vi "CAN_Send Diag Message.vi"(0 "Write Session in":refnum<k21>, 1 "Enum":T2=enum."Get Calibration Status", 2 "Postion":u16=3, 4 "ECU Info in":T1, 5 "Read Session in":refnum<k21>, 7 "ODX File Path":path=path "C:/LegacyApp/DB_0CA_7100_4M0_0004_73710BVW3710/DB_0CA_7100_4M0_0004_73710BVW3710/DB_0CA_7100_4M0_0004_73710BVW3710.odx", 8 "Tester":refnum<k21>, 9 "Tx Msg":u8[](array[numeric])=[2, 26, 156, 255, 255, 255, 255, 255] format="%02x", 11 "error in (no error)":errorcluster, 12 "Download CAL Progress":refnum<vi>, 13 "Download CAL Time":refnum<vi>) -> (6 "ECU Info":T1, 10 "TxRx Data":string[][](array[string]), 14 "Response Good?":bool, 15 "error out":errorcluster)   [LabVIEW 2014]
uses:
  Diagnostic Message.ctl
  <vilib>/xnet/xnet.llb/XNET Frame CAN.ctl
  <vilib>/xnet/xnet.llb/XNET Frame Type CAN.ctl
  CAN Communication VI's/Typedefs/Select Session.ctl
  typedefs/All Motions.ctl
  <vilib>/xnet/xnet.llb/XNET Write (Frame CAN).vi
  <vilib>/xnet/xnet.llb/XNET Read (Frame CAN).vi
panel:
  out "Rx Message":u8[](array[numeric]) format="%02x"
  out "Error String Out":string
  in  "Tx Arbitration Id":u32=402391172 format="%.0x"
  out "Part Number":string
  out "Vehicle Type":string
  out "SW level":string
  out "Calibrated":bool
  out "HW level":string
  out "CAL level":string
  out "Boot level":string
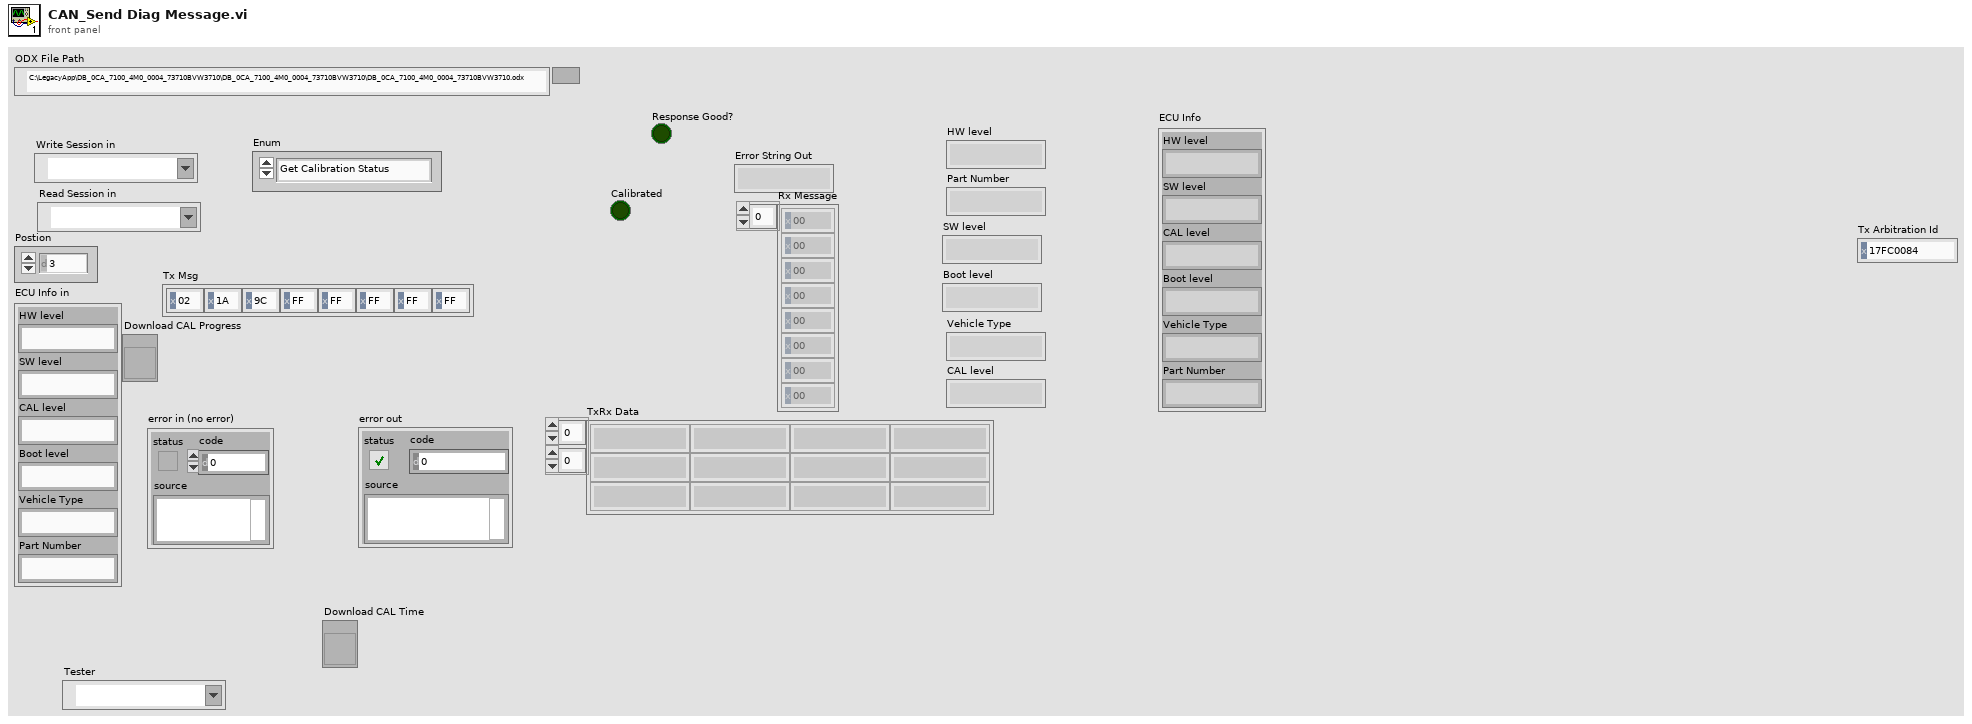
[diagram p1: front panel]
types:
  T1 = cluster{"HW level":string, "SW level":string, "CAL level":string, "Boot level":string, "Vehicle Type":string, "Part Number":string}
  T2 = typedef "Diagnostic Message.ctl" = enum16{"User Select", "Get User Multi-Frame", "Diag Session Prog", "Diag Session Ext", "Diag Session EOL", "Diag Session Default", "Diag Session Dev", "Read Active Session", "Read HW", "Read SW", "Read Part Number", "Learn Start Glass", "Learn Start Rollo", "Get Calibration Status", "Read SW CAL Boot", "Go to Position", "Get Parametric Mode Status", "Enable Parametric Mode", "Disable Parametric Mode", "Enable Production Mode", "Disable Production Mode", "Reset ECU", "Go to Slide Close", "Go to Slide Open", "Go to Vent Open", "Rollo Open", "Rollo Close", "Write Vehicle Type", "Read Vehicle Type", "Clear DTC", "Check Teach DTC", "Write Shop Code", "Download CAL"}
  T3 = typedef "XNET Frame CAN.ctl" = cluster{"timestamp":timestamp, "payload":u8[], "identifier":u32, "type":T4, "extended?":bool, "echo?":bool}
  T4 = typedef "XNET Frame Type CAN.ctl" = u8
  T5 = typedef "Select Session.ctl" = enum16{"DefaultSession", "Development", "Extended", "EOL", "Programming"}
  T6 = typedef "All Motions.ctl" = enum16{"Idle", "Glass Teach", "Glass Slide Open", "Glass Slide Open 2", "Glass Slide Close", "Glass Slide Close 2", "Glass Vent Open", "Glass Vent Close", "Sunshade Teach", "Sunshade Teach 2", "Sunshade Open", "Sunshade Open 2", "Sunshade Close", "Sunshade Close 2", "Glass Slide Open Sunshade Open", "Glass Slide Open 2 Sunshade Open", "Glass Slide Open Sunshade Close", "Glass Slide Open 2 Sunshade Close", "Glass Slide Close Sunshade Open", "Glass Slide Close 2 Sunshade Open", "Glass Slide Close Sunshade Close", "Glass Slide Close 2 Sunshade Close", "Glass Vent Open Sunshade Open", "Glass Vent Open Sunshade Close", "Glass Vent Close Sunshade Open", "Glass Vent Close Sunshade Close", "Express Glass Slide Open", "Express Glass Slide Open 2", "Express Glass Slide Close", "Express Glass Slide Close 2", "Express Glass Vent Open", "Express Glass Vent Close", "Express Sunshade Open", "Express Sunshade Close", "Express Sunshade Open 2", "Express Sunshade Close 2", "Express Glass Slide Open Sunshade Open", "Express Glass Slide Open 2 Sunshade Open", "Express Glass Slide Open Sunshade Close", "Express Glass Slide Open 2 Sunshade Close", "Express Glass Slide Close Sunshade Open", "Express Glass Slide Close 2 Sunshade Open", "Express Glass Slide Close Sunshade Close", "Express Glass Slide Close 2 Sunshade Close", "Express Glass Vent Open Sunshade Open", "Express Glass Vent Open Sunshade Close", "Express Glass Vent Close Sunshade Open", "Express Glass Vent Close Sunshade Close", "Goto Position Glass", "Goto Position Sunshade"}
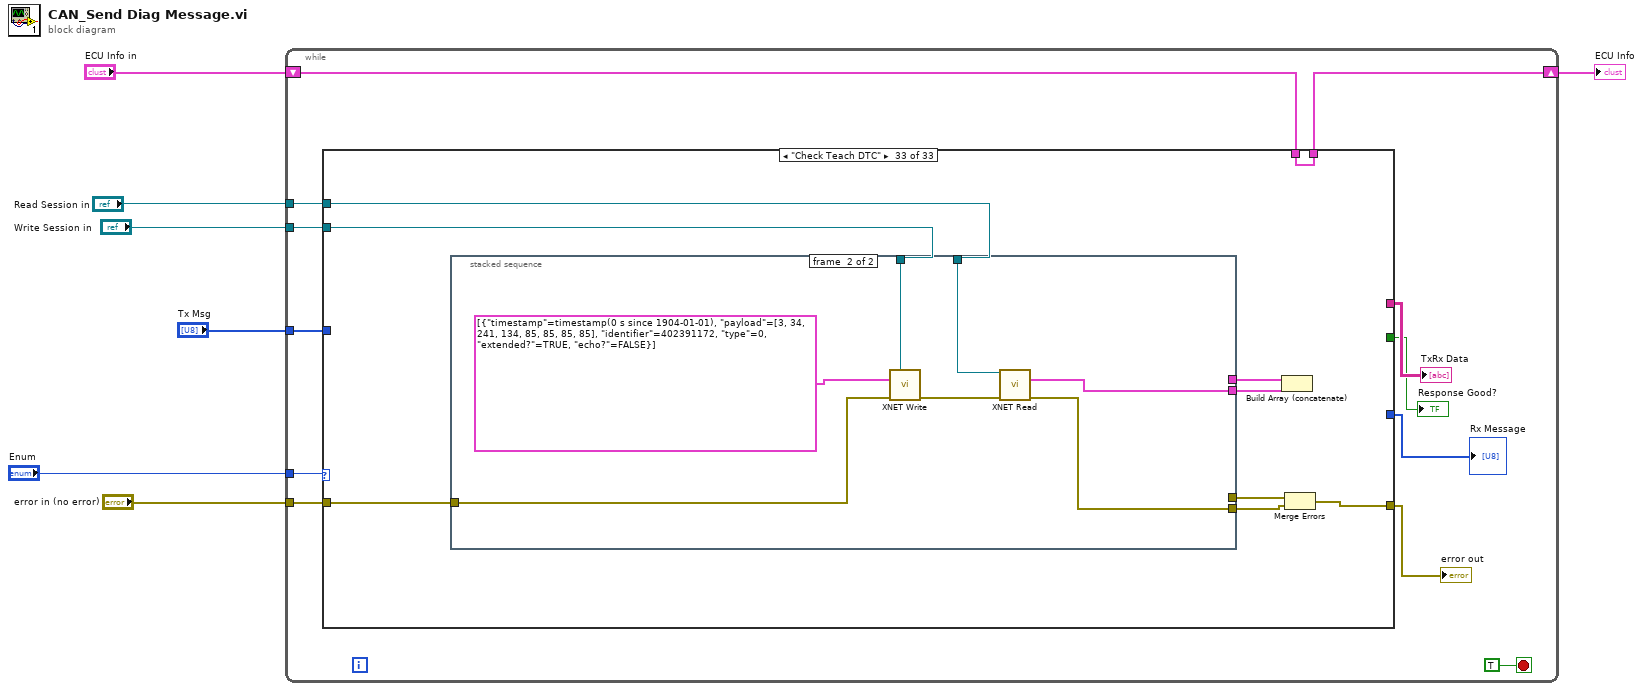
[diagram p0: block diagram]
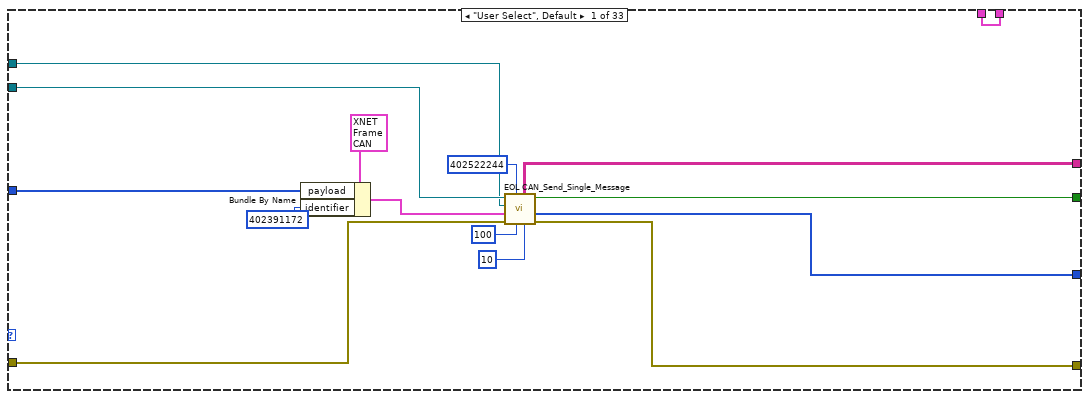
[diagram p2: hidden frame]
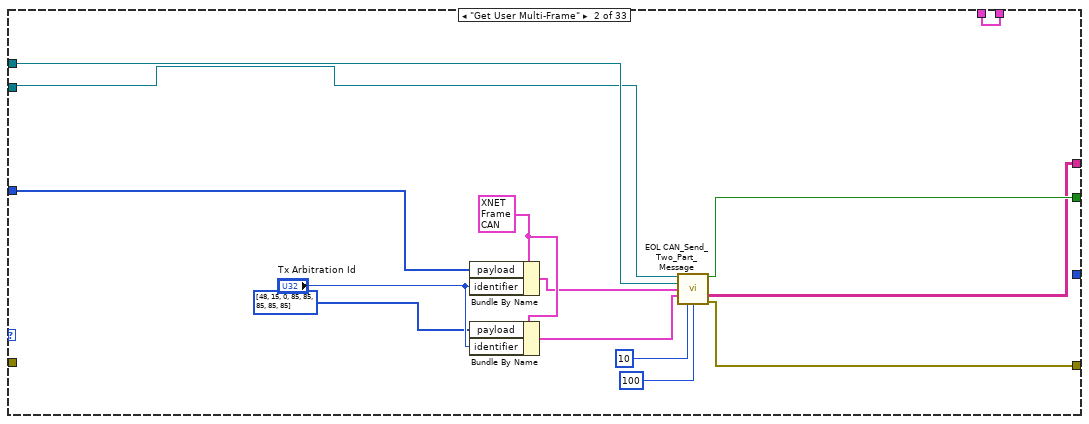
[diagram p3: hidden frame]
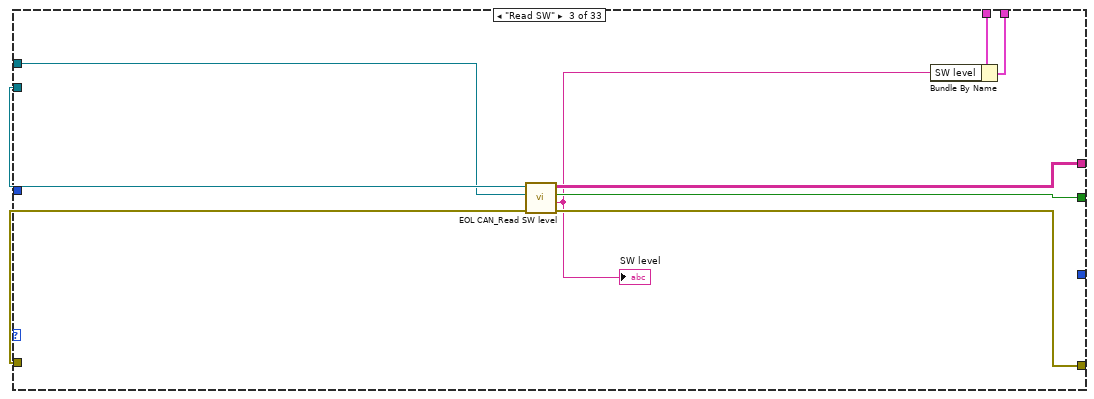
[diagram p4: hidden frame]
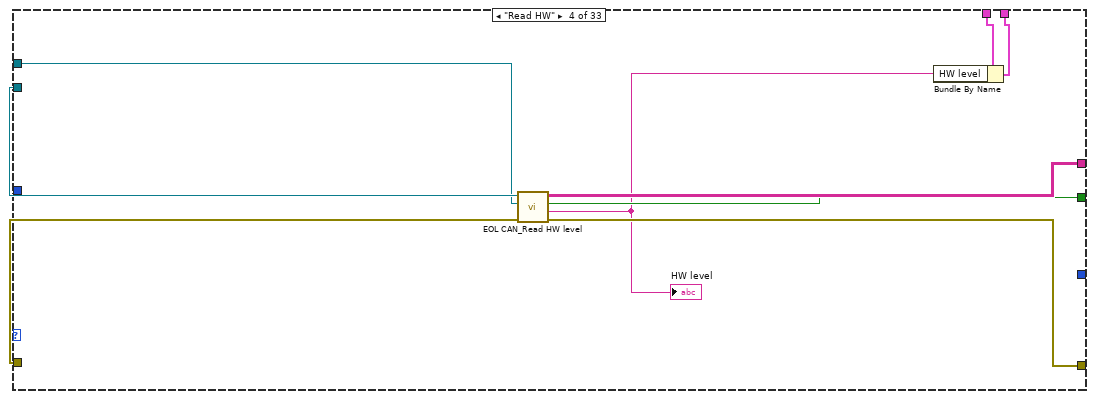
[diagram p5: hidden frame]
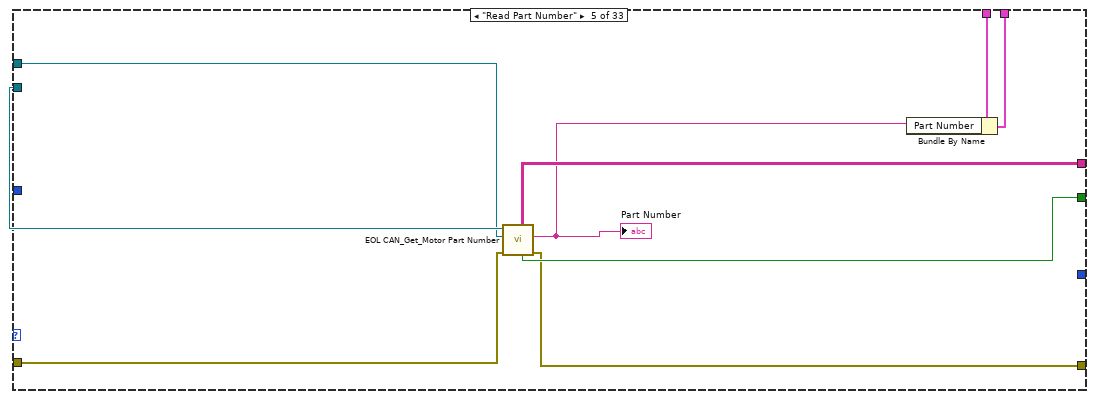
[diagram p6: hidden frame]
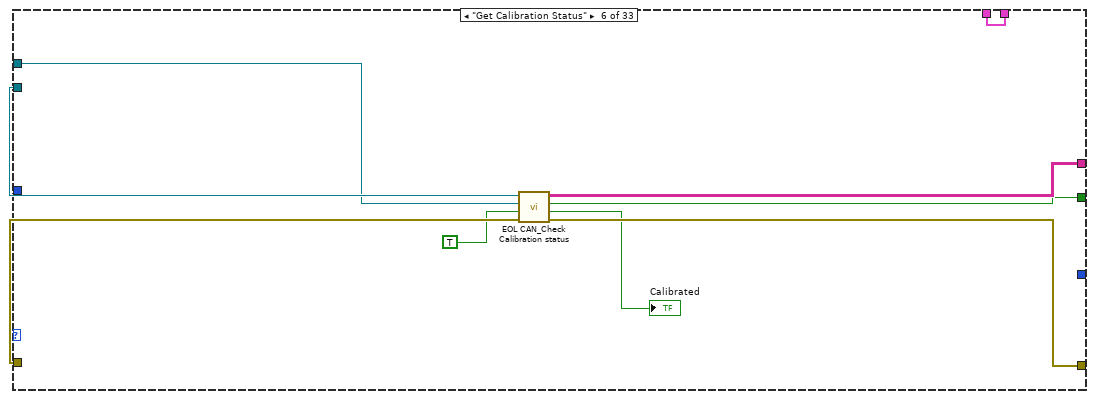
[diagram p7: hidden frame]
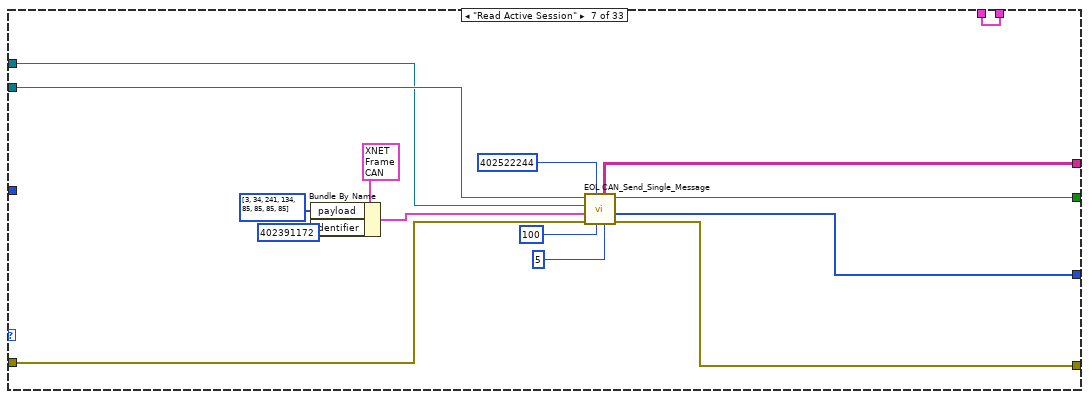
[diagram p8: hidden frame]
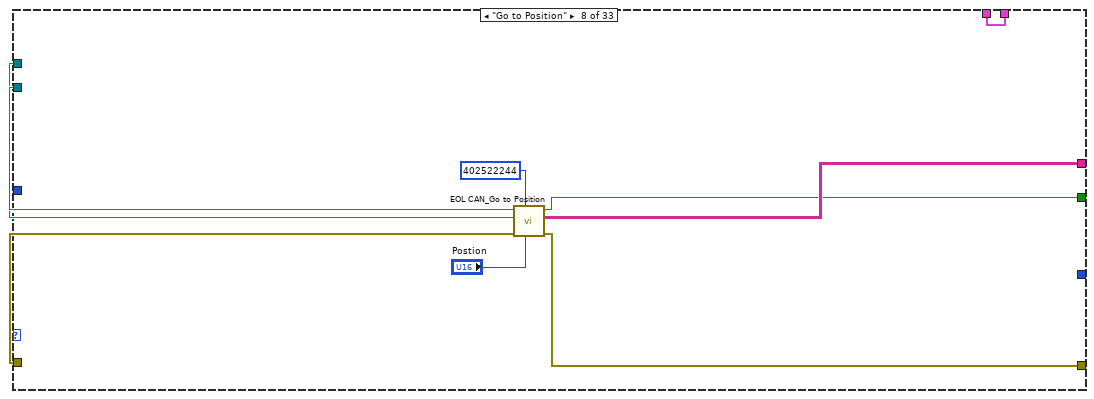
[diagram p9: hidden frame]
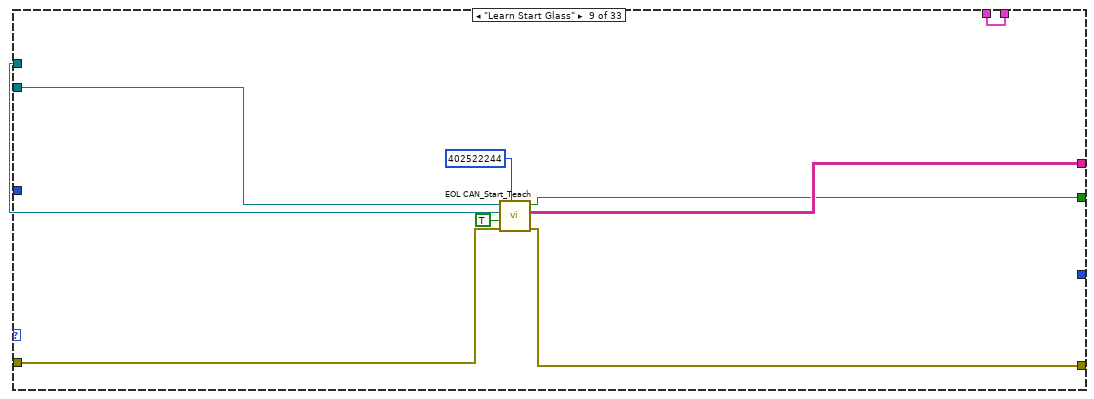
[diagram p10: hidden frame]
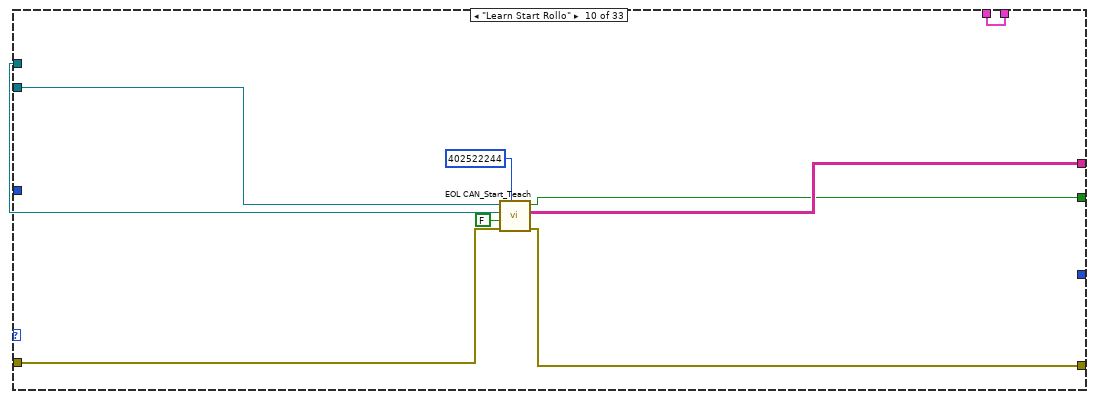
[diagram p11: hidden frame]
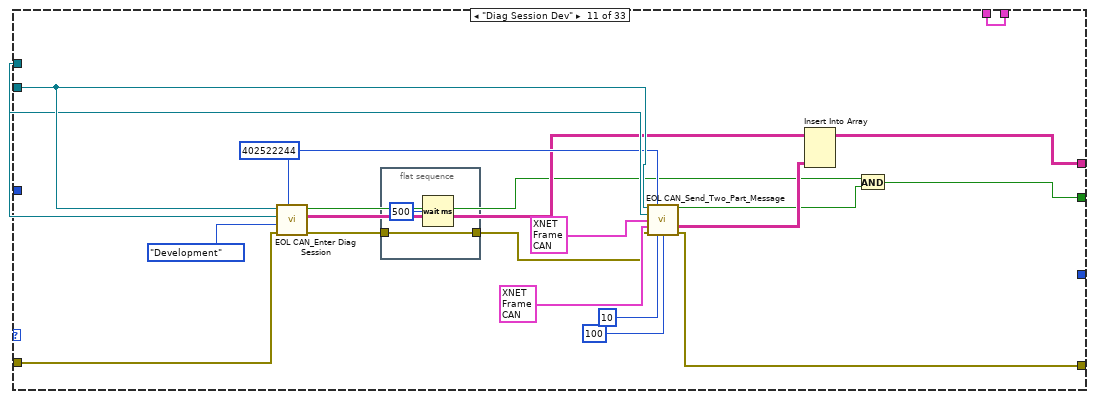
[diagram p12: hidden frame]
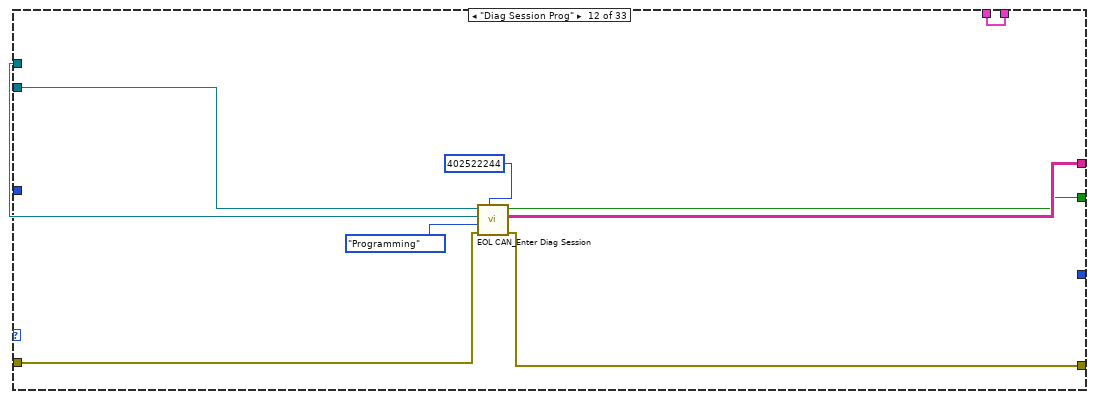
[diagram p13: hidden frame]
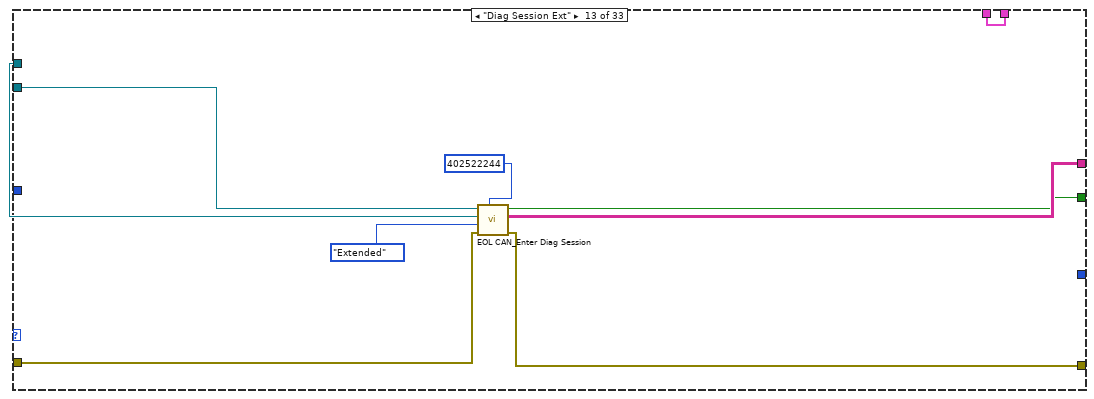
[diagram p14: hidden frame]
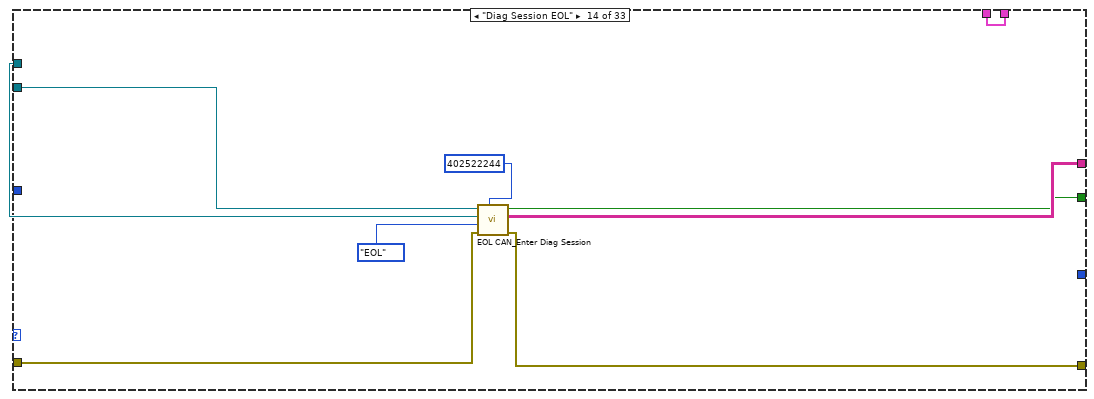
[diagram p15: hidden frame]
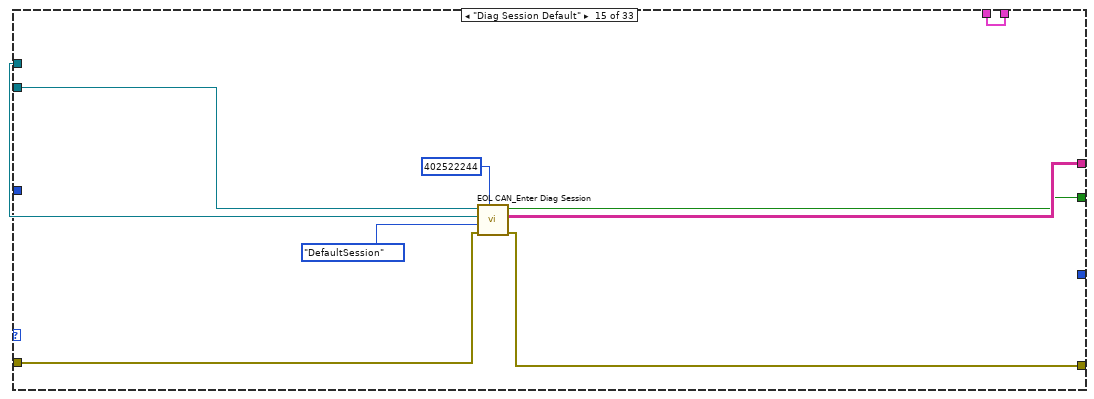
[diagram p16: hidden frame]
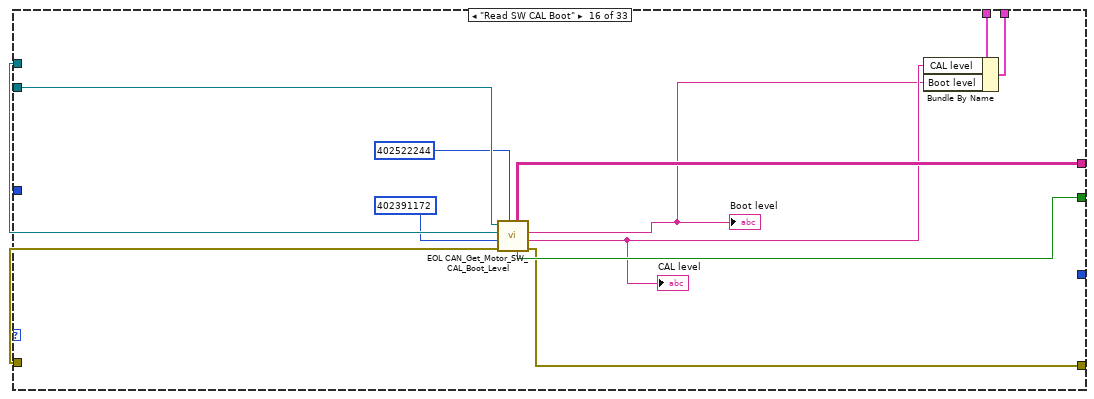
[diagram p17: hidden frame]
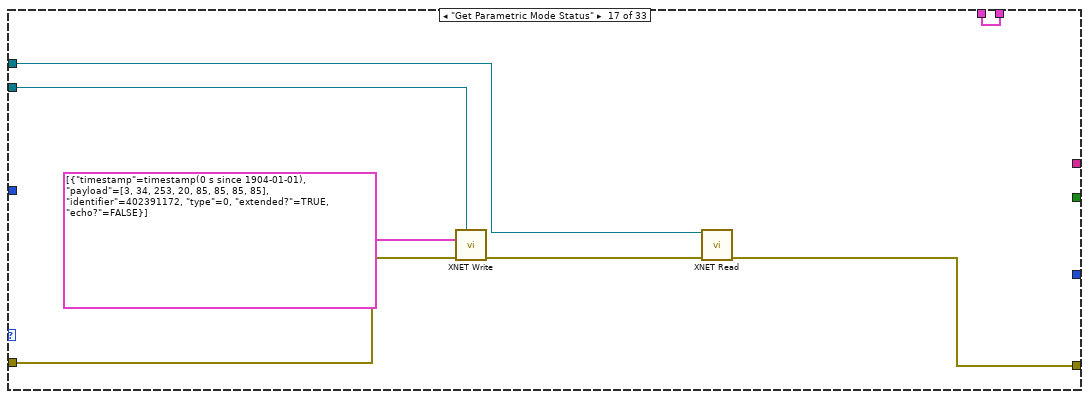
[diagram p18: hidden frame]
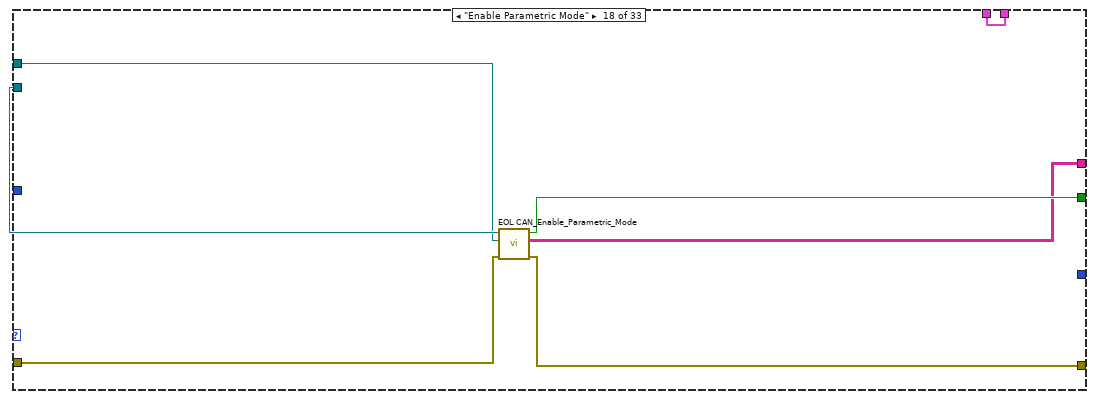
[diagram p19: hidden frame]
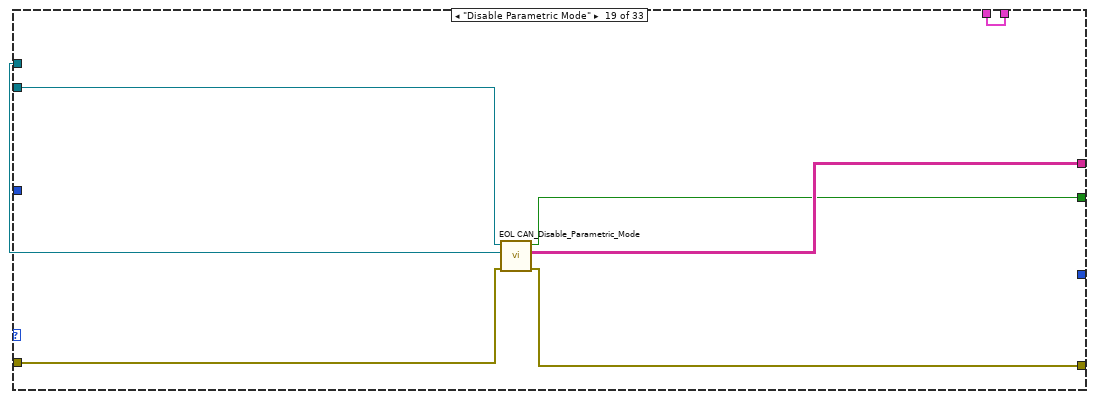
[diagram p20: hidden frame]
diagram:
  n1 = while {
    tunnel: "error in (no error)" -> [w19]
    tunnel: "Read Session in" -> [w17]
    tunnel: "Write Session in" -> [w16]
    tunnel: "Enum" -> [w15]
    shift-right: [w11] -> w3
    shift-left: "ECU Info in" -> [w10]
    tunnel: "Tx Msg" -> [w9]
    stop <- TRUE stop-if-true
    n2 = case shown="\"Check Teach DTC\"" w15 {
      tunnel: w17 -> [w33 w40 w52 w61 w73 w83 w98 w105 w115 w124 w141 w150 w159 w168 w177 w193 w200 w207 w211 w221 w228 w236 w245 w254 w263 w272 w281 w284 w291 w305 w319 w325 w334]
      tunnel: w16 -> [w34 w39 w53 w62 w74 w84 w99 w106 w116 w125 w143 w151 w160 w169 w178 w194 w202 w208 w212 w222 w229 w237 w246 w255 w264 w273 w282 w285 w292 w306 w318 w326 w336]
      tunnel: w19 -> [w32 _ w57 w66 w75 w82 w97 w108 w117 w126 w145 w156 w165 w174 w183 w195 w201 w209 w216 w223 w230 w238 w247 w256 w265 w274 w283 _ _ _ w320 w327 w335]
      tunnel: [w31 w35 w56 w65 w70 w81 w96 w107 w113 w122 w142 w155 w164 w173 w182 w188 w197 w204 w215 w218 w225 w232 w241 w250 w259 w268 w277 w288 w295 errorcluster {"status"=FALSE, "code"=0, "source"=""} ("error IO") w313 w324 w333] -> w18
      tunnel: [w30 w36 w55 w64 w72 w80 w95 w103 w112 w121 w135 w154 w163 w172 w181 w190 _ w205 w214 w219 w226 w234 w242 w251 w260 w269 w278 w289 w296 w301 w315 w322 _] -> w14
      tunnel: [w29 w37 w54 w63 w71 w77 w94 w102 w111 w120 w132 w153 w162 w171 w180 w189 _ w206 w213 w220 w227 w233 w243 w252 w261 w270 w279 w287 w294 w298 w314 w323 _] -> w13
      tunnel: [w28 _ _ _ _ _ w91 _ _ _ _ _ _ _ _ _ _ _ _ _ _ _ _ _ _ _ _ w286 w293 _ _ _ _] -> w8
      tunnel: [w21 w48 w50 w58 w68 w76 w85 w100 w110 w119 w127 w148 w157 w166 w175 w186 w196 w203 w210 w217 w224 w231 w239 w248 w257 w266 w275 w290 w297 w309 w311 w321 w328] -> w11
      tunnel: w10 -> [w21 w48 w51 w59 w67 w76 w85 w100 w110 w119 w127 w148 w157 w166 w175 w187 w196 w203 w210 w217 w224 w231 w239 w248 w257 w266 w275 w290 w297 w309 w312 w321 w328]
      tunnel: w9 -> [w20 w38 _ _ _ _ _ _ _ _ _ _ _ _ _ _ _ _ _ _ _ _ _ _ _ _ _ _ _ _ _ _ _]
      frame "User Select", Default {
        n3 = Bundle By Name(cluster=T3 {"timestamp"=timestamp(0 s since 1904-01-01), "payload"=[2, 39, 3, 85, 85, 85, 85, 85], "identifier"=402391172, "type"=0, "extended?"=TRUE, "echo?"=FALSE} ("Tx CAN frame"), "payload"=w20, "identifier"=u32 402391172) -> (w26:T3)
        n4 = call "EOL CAN_Send_Single_Message.vi"("Retries"=10, "Msg Wait Time"=u32 100, "Rx Arbitration Id"=u32 402522244, "Error in"=w32, "Tx CAN frame"=w26, "Read Session in"=w33, "Write Session in"=w34) -> ("Error out"=w31:errorcluster, "Rx Message"=w28:u8[], "Response Good?"=w29:bool, "TxRx Data"=w30:string[][])  [unwired: 1 out]
      }
      frame "Get User Multi-Frame" {
        w42 = T3 {"timestamp"=timestamp(0 s since 1904-01-01), "payload"=[2, 39, 3, 85, 85, 85, 85, 85], "identifier"=402391172, "type"=0, "extended?"=TRUE, "echo?"=FALSE} ("Tx CAN frame 1")
        n5 = Bundle By Name(cluster=w42, "payload"=w38, "identifier"="Tx Arbitration Id") -> (w41:T3)
        n6 = Bundle By Name(cluster=w42, "payload"=u8[] [48, 15, 0, 85, 85, 85, 85, 85] ("Transmit Data"), "identifier"="Tx Arbitration Id") -> (w43:T3)
        n7 = call "EOL CAN_Send_Two_Part_Message.vi"("Write Session in"=w39, "Read Session in"=w40, "Tx CAN frame 1"=w41, "Tx CAN frame 2"=w43, "Retries"=10, "Msg Wait Time"=u32 100) -> ("Response Good?"=w37:bool, "TxRx Data"=w36:string[][], "error out"=w35:errorcluster)  [unwired: 6 in, 1 out]
      }
      frame "Read SW" {
        n8 = call "EOL CAN_Read SW level.vi"("error in (no error)"=w57, "Read Session in"=w52, "Write Session in"=w53) -> ("error out"=w56:errorcluster, "SW level"=w49:string, "Response Good?"=w54:bool, "TxRx Data"=w55:string[][])  [unwired: 5 in]
        "SW level" <- w49
        n9 = Bundle By Name(cluster=w51, "SW level"=w49) -> (w50:T1)
      }
      frame "Read HW" {
        n10 = call "EOL CAN_Read HW level.vi"("error in (no error)"=w66, "Read Session in"=w61, "Write Session in"=w62) -> ("error out"=w65:errorcluster, "HW level"=w60:string, "Response Good?"=w63:bool, "TxRx Data"=w64:string[][])  [unwired: 5 in]
        "HW level" <- w60
        n11 = Bundle By Name(cluster=w59, "HW level"=w60) -> (w58:T1)
      }
      frame "Read Part Number" {
        n12 = call "EOL CAN_Get_Motor Part Number.vi"("error in (no error)"=w75, "Read Session in"=w73, "Write Session in"=w74) -> ("error out"=w70:errorcluster, "Part Number"=w69:string, "Response Good?"=w71:bool, "TxRx Data"=w72:string[][])  [unwired: 5 in]
        "Part Number" <- w69
        n13 = Bundle By Name(cluster=w67, "Part Number"=w69) -> (w68:T1)
      }
      frame "Get Calibration Status" {
        n14 = call "EOL CAN_Check Calibration status.vi"("error in (no error)"=w82, "Glass?"=TRUE, "Read Session in"=w83, "Write Session in"=w84) -> ("error out"=w81:errorcluster, "Calibrated"=→"Calibrated":bool, "Response Good?"=w77:bool, "TxRx Data"=w80:string[][])  [unwired: 4 in]
      }
      frame "Read Active Session" {
        n15 = Bundle By Name(cluster=T3 {"timestamp"=timestamp(0 s since 1904-01-01), "payload"=[2, 39, 3, 85, 85, 85, 85, 85], "identifier"=402391172, "type"=0, "extended?"=TRUE, "echo?"=FALSE} ("Tx CAN frame"), "payload"=u8[] [3, 34, 241, 134, 85, 85, 85, 85], "identifier"=u32 402391172) -> (w88:T3)
        n16 = call "EOL CAN_Send_Single_Message.vi"("Retries"=5, "Msg Wait Time"=u32 100, "Rx Arbitration Id"=u32 402522244, "Error in"=w97, "Tx CAN frame"=w88, "Read Session in"=w98, "Write Session in"=w99) -> ("Error out"=w96:errorcluster, "Rx Message"=w91:u8[], "Response Good?"=w94:bool, "TxRx Data"=w95:string[][])  [unwired: 1 out]
      }
      frame "Go to Position" {
        n17 = call "EOL CAN_Go to Position.vi"("Postion"="Postion", "Rx Arbitration Id"=u32 402522244, "Error in"=w108, "Read Session in"=w105, "Write Session in"=w106) -> ("Error out"=w107:errorcluster, "TxRx Data"=w103:string[][], "Response Good?"=w102:bool)  [unwired: 4 in]
      }
      frame "Learn Start Glass" {
        n18 = call "EOL CAN_Start_Teach.vi"("Rx Arbitration Id"=u32 402522244, "Error in"=w117, "Glass?"=TRUE, "Read Session in"=w115, "Write Session in"=w116) -> ("Error out"=w113:errorcluster, "TxRx Data"=w112:string[][], "Response Good?"=w111:bool)  [unwired: 4 in]
      }
      frame "Learn Start Rollo" {
        n19 = call "EOL CAN_Start_Teach.vi"("Rx Arbitration Id"=u32 402522244, "Error in"=w126, "Glass?"=FALSE, "Read Session in"=w124, "Write Session in"=w125) -> ("Error out"=w122:errorcluster, "TxRx Data"=w121:string[][], "Response Good?"=w120:bool)  [unwired: 4 in]
      }
      frame "Diag Session Dev" {
        w140 = u32 402522244 ("Rx Arbitration Id")
        n20 = call "EOL CAN_Enter Diag Session.vi"("Rx Arbitration Id"=w140, "Error in"=w145, "Session"=Select_Session."Development", "Read Session in"=w141, "Write Session in"=w143) -> ("Error out"=w131:errorcluster, "TxRx Data"=w137:string[][], "Response Good?"=w133:bool)  [unwired: 4 in]
        n21 = flat-sequence {
          tunnel: w131 -> [w146]
          tunnel: [w146] -> w130
          frame #0 {
            n22 = Wait (ms)(milliseconds to wait=u32 500) -> ()  [unwired: 1 out]
          }
        }
        n23 = call "EOL CAN_Send_Two_Part_Message.vi"("Write Session in"=w143, "Rx Arbitration Id"=w140, "Read Session in"=w141, "Tx CAN frame 1"=T3 {"timestamp"=timestamp(0 s since 1904-01-01), "payload"=[3, 34, 254, 253, 85, 85, 85, 85], "identifier"=402391172, "type"=8, "extended?"=TRUE, "echo?"=FALSE}, "Tx CAN frame 2"=T3 {"timestamp"=timestamp(0 s since 1904-01-01), "payload"=[48, 15, 0, 85, 85, 85, 85, 85], "identifier"=402391172, "type"=8, "extended?"=TRUE, "echo?"=FALSE}, "error in (no error)"=w130, "Retries"=10, "Msg Wait Time"=u32 100) -> ("Response Good?"=w134:bool, "TxRx Data"=w136:string[][], "error out"=w142:errorcluster)  [unwired: 4 in, 1 out]
        n24 = Insert Into Array(array=w137, new element=w136) -> (w135:string[][])  [unwired: 2 in]
        n25 = And(x=w133, y=w134) -> (x .and. y?=w132:bool)
      }
      frame "Diag Session Prog" {
        n26 = call "EOL CAN_Enter Diag Session.vi"("Rx Arbitration Id"=u32 402522244, "Error in"=w156, "Session"=Select_Session."Programming", "Read Session in"=w150, "Write Session in"=w151) -> ("Error out"=w155:errorcluster, "TxRx Data"=w154:string[][], "Response Good?"=w153:bool)  [unwired: 4 in]
      }
      frame "Diag Session Ext" {
        n27 = call "EOL CAN_Enter Diag Session.vi"("Rx Arbitration Id"=u32 402522244, "Error in"=w165, "Session"=Select_Session."Extended", "Read Session in"=w159, "Write Session in"=w160) -> ("Error out"=w164:errorcluster, "TxRx Data"=w163:string[][], "Response Good?"=w162:bool)  [unwired: 4 in]
      }
      frame "Diag Session EOL" {
        n28 = call "EOL CAN_Enter Diag Session.vi"("Rx Arbitration Id"=u32 402522244, "Error in"=w174, "Session"=Select_Session."EOL", "Read Session in"=w168, "Write Session in"=w169) -> ("Error out"=w173:errorcluster, "TxRx Data"=w172:string[][], "Response Good?"=w171:bool)  [unwired: 4 in]
      }
      frame "Diag Session Default" {
        n29 = call "EOL CAN_Enter Diag Session.vi"("Rx Arbitration Id"=u32 402522244, "Error in"=w183, "Session"=Select_Session."DefaultSession", "Read Session in"=w177, "Write Session in"=w178) -> ("Error out"=w182:errorcluster, "TxRx Data"=w181:string[][], "Response Good?"=w180:bool)  [unwired: 4 in]
      }
      frame "Read SW CAL Boot" {
        n30 = call "EOL CAN_Get_Motor_SW_CAL_Boot_Level.vi"("Rx Arbitration Id"=u32 402522244, "error in (no error)"=w195, "Tx Arbitration Id"=u32 402391172 ("identifier"), "Read Session in"=w193, "Write Session in"=w194) -> ("error out"=w188:errorcluster, "CAL level"=w185:string, "Boot level"=w184:string, "Response Good?"=w189:bool, "TxRx Data"=w190:string[][])  [unwired: 1 in, 1 out]
        "Boot level" <- w184
        "CAL level" <- w185
        n31 = Bundle By Name(cluster=w187, "CAL level"=w185, "Boot level"=w184) -> (w186:T1)
      }
      frame "Get Parametric Mode Status" {
        n32 = call-poly <vilib>:"XNET Write.vi"("session in"=w202, "data"=T3[] [{"timestamp"=timestamp(0 s since 1904-01-01), "payload"=[3, 34, 253, 20, 85, 85, 85, 85], "identifier"=402391172, "type"=0, "extended?"=TRUE, "echo?"=FALSE}] ("Frame to Send 2"), "error in (no error)"=w201) -> ("error out"=w198:errorcluster)  [unwired: 11 in, 1 out]
        n33 = call-poly <vilib>:"XNET Read.vi"("session in"=w200, "error in (no error)"=w198) -> ("error out"=w197:errorcluster)  [unwired: 10 in, 3 out]
      }
      frame "Enable Parametric Mode" {
        n34 = call "EOL CAN_Enable_Parametric_Mode.vi"("Error in"=w209, "Read Session in"=w207, "Write Session in"=w208) -> ("Error out"=w204:errorcluster, "debug log"=w205:string[][], "Response Good?"=w206:bool)  [unwired: 6 in]
      }
      frame "Disable Parametric Mode" {
        n35 = call "EOL CAN_Disable_Parametric_Mode.vi"("Error in"=w216, "Read Session in"=w211, "Write Session in"=w212) -> ("Error out"=w215:errorcluster, "debug log"=w214:string[][], "Response Good?"=w213:bool)  [unwired: 6 in]
      }
      frame "Enable Production Mode" {
        n36 = call "EOL CAN_Enable_Production_Mode.vi"("Error in"=w223, "Read Session in"=w221, "Write Session in"=w222) -> ("Error out"=w218:errorcluster, "debug log"=w219:string[][], "Response Good?"=w220:bool)  [unwired: 6 in]
      }
      frame "Disable Production Mode" {
        n37 = call "EOL CAN_Disable_Production_Mode.vi"("Error in"=w230, "Read Session in"=w228, "Write Session in"=w229) -> ("Error out"=w225:errorcluster, "debug log"=w226:string[][], "Response Good?"=w227:bool)  [unwired: 6 in]
      }
      frame "Reset ECU" {
        n38 = call "EOL CAN_Reset ECU.vi"("Rx Arbitration Id"=u32 402522244, "Error in"=w238, "Read Session in"=w236, "Write Session in"=w237) -> ("Error out"=w232:errorcluster, "Response Good?"=w233:bool, "TxRx Data"=w234:string[][])  [unwired: 5 in]
      }
      frame "Go to Slide Close" {
        n39 = call "EOL CAN_Target Motion.vi"("Rx Arbitration Id"=u32 402522244, "Error in"=w247, "All Motions"=All_Motions."Glass Slide Close", "Read Session in"=w245, "Write Session in"=w246) -> ("Error out"=w241:errorcluster, "TxRx Data"=w242:string[][], "Response Good?"=w243:bool)  [unwired: 4 in]
      }
      frame "Go to Slide Open" {
        n40 = call "EOL CAN_Target Motion.vi"("Rx Arbitration Id"=u32 402522244, "Error in"=w256, "All Motions"=All_Motions."Glass Slide Open", "Read Session in"=w254, "Write Session in"=w255) -> ("Error out"=w250:errorcluster, "TxRx Data"=w251:string[][], "Response Good?"=w252:bool)  [unwired: 4 in]
      }
      frame "Go to Vent Open" {
        n41 = call "EOL CAN_Target Motion.vi"("Rx Arbitration Id"=u32 402522244, "Error in"=w265, "All Motions"=All_Motions."Glass Vent Open", "Read Session in"=w263, "Write Session in"=w264) -> ("Error out"=w259:errorcluster, "TxRx Data"=w260:string[][], "Response Good?"=w261:bool)  [unwired: 4 in]
      }
      frame "Rollo Open" {
        n42 = call "EOL CAN_Target Motion.vi"("Rx Arbitration Id"=u32 402522244, "Error in"=w274, "All Motions"=All_Motions."Sunshade Open", "Read Session in"=w272, "Write Session in"=w273) -> ("Error out"=w268:errorcluster, "TxRx Data"=w269:string[][], "Response Good?"=w270:bool)  [unwired: 4 in]
      }
      frame "Rollo Close" {
        n43 = call "EOL CAN_Target Motion.vi"("Rx Arbitration Id"=u32 402522244, "Error in"=w283, "All Motions"=All_Motions."Sunshade Close", "Read Session in"=w281, "Write Session in"=w282) -> ("Error out"=w277:errorcluster, "TxRx Data"=w278:string[][], "Response Good?"=w279:bool)  [unwired: 4 in]
      }
      frame "Write Vehicle Type" {
        n44 = call "EOL CAN_Write Vehicle Type.vi"("Read Session in"=w284, "Write Session in"=w285) -> ("error out"=w288:errorcluster, "Rx Message"=w286:u8[], "Response Good?"=w287:bool, "Array"=w289:string[][])  [unwired: 6 in]
      }
      frame "Write Shop Code" {
        n45 = call "EOL CAN_Write Repair Shop Code.vi"("Read Session in"=w291, "Write Session in"=w292) -> ("error out"=w295:errorcluster, "Rx Message"=w293:u8[], "Response Good?"=w294:bool, "TxRxData"=w296:string[][])  [unwired: 6 in]
      }
      frame "Download CAL" {
        n46 = call "EOL CAN_Download CAL.vi"("Download CAL Progress"="Download CAL Progress", "Download CAL Time"="Download CAL Time", "ODX File Path"="ODX File Path", "Tester"="Tester", "Glass?"=TRUE, "Read Session in"=w305, "DSC Write Session in"=w306) -> ("Error String Out"=→"Error String Out":string, "TxRx Data"=w301:string[][], "Response Good?"=w298:bool)  [unwired: 2 in]
      }
      frame "Read Vehicle Type" {
        n47 = call "EOL CAN_Get Vehicle type.vi"("Rx Arbitration Id"=u32 402522244, "error in (no error)"=w320, "Tx Arbitration Id"=u32 402391172, "Read Session in"=w319, "Write Session in"=w318) -> ("error out"=w313:errorcluster, "Vehicle Type"=w310:string, "Response Good?"=w314:bool, "TxRx Data"=w315:string[][])  [unwired: 3 in]
        "Vehicle Type" <- w310
        n48 = Bundle By Name(cluster=w312, "Vehicle Type"=w310) -> (w311:T1)
      }
      frame "Clear DTC" {
        n49 = call "EOL CAN_Clear_DTC's.vi"("Error in"=w327, "Read Session in"=w325, "Write Session in"=w326) -> ("Error out"=w324:errorcluster, "TxRx Data"=w322:string[][], "Response Good?"=w323:bool)  [unwired: 6 in]
      }
      frame "Check Teach DTC" {
        n50 = stacked-sequence {
          tunnel: w336 -> [w344 w352]
          tunnel: w335 -> [w343 w351]
          tunnel: [w341 _] -> w332
          tunnel: w334 -> [w342 w350]
          tunnel: [w340 _] -> w330
          tunnel: [_ w349] -> w329
          tunnel: [_ w348] -> w331
          frame #0 {
            n51 = call-poly <vilib>:"XNET Write.vi"("session in"=w344, "data"=T3[] [{"timestamp"=timestamp(0 s since 1904-01-01), "payload"=[2, 16, 79, 85, 85, 85, 85, 85], "identifier"=402391172, "type"=0, "extended?"=TRUE, "echo?"=FALSE}] ("Frame to Send 2"), "error in (no error)"=w343) -> ("error out"=w338:errorcluster)  [unwired: 11 in, 1 out]
            n52 = call "Time Delay22"("error in (no error)"=w338, "Delay Time (s)"=0.05) -> ("error out"=w337:errorcluster)  [unwired: 9 in]
            n53 = call-poly <vilib>:"XNET Read.vi"("session in"=w342, "error in (no error)"=w337) -> ("data"=w340:T3[], "error out"=w341:errorcluster)  [unwired: 10 in, 2 out]
          }
          frame #1 {
            n54 = call-poly <vilib>:"XNET Write.vi"("session in"=w352, "data"=T3[] [{"timestamp"=timestamp(0 s since 1904-01-01), "payload"=[3, 34, 241, 134, 85, 85, 85, 85], "identifier"=402391172, "type"=0, "extended?"=TRUE, "echo?"=FALSE}] ("Frame to Send 2"), "error in (no error)"=w351) -> ("error out"=w347:errorcluster)  [unwired: 11 in, 1 out]
            n55 = call-poly <vilib>:"XNET Read.vi"("session in"=w350, "error in (no error)"=w347) -> ("data"=w349:T3[], "error out"=w348:errorcluster)  [unwired: 10 in, 2 out]
          }
        }
        n56 = Build Array (concatenate)(w330, w329) -> ()  [unwired: 1 out]
        n57 = Merge Errors(w332, w331) -> (w333:errorcluster)
      }
    }
    "error out" <- w18
    "TxRx Data" <- w14
    "Response Good?" <- w13
    "Rx Message" <- w8
  }
  "ECU Info" <- w3
